vi "DRWMresult.vi"(7 "价值曲线":cluster{"棒位积累":dbl[], dbl[]}[](array[cluster]), 8 "下段总价值":dbl, 9 "上段总价值":dbl, 10 "下段正反应性":dbl, 11 "上段正反应性":dbl) -> ()   [LabVIEW 2020]
panel:
  out "下段测量总价值":dbl
  out "上段测量总价值":dbl
  out "下段降棒前正反应性":dbl
  out "上段降棒前正反应性":dbl
  out "棒价值曲线":cluster{"棒位积累":dbl[], dbl[]}[](graph) caption="XY Graph - Dark"
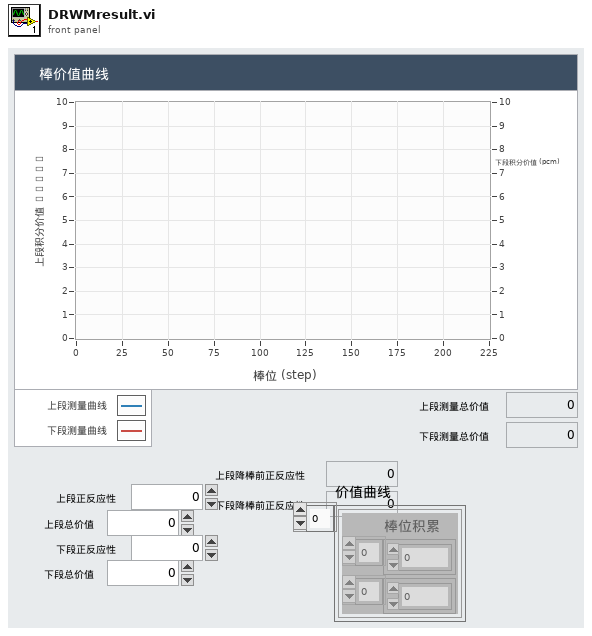
[diagram p1: front panel]
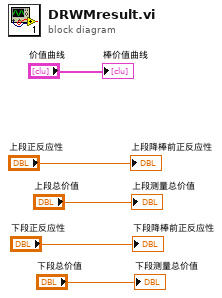
[diagram p0: block diagram]
diagram:
  "棒价值曲线" <- "价值曲线"
  "上段降棒前正反应性" <- "上段正反应性"
  "下段降棒前正反应性" <- "下段正反应性"
  "上段测量总价值" <- "上段总价值"
  "下段测量总价值" <- "下段总价值"
